vi "FindAllChildrenOf.vi"(10 "Name":string, 11 "RelationshipBrowser":refnum<class "Relationships.lvclass">) -> (3 "Children":refnum<class "Person.lvclass">[](array[class]))   [LabVIEW 2018, in "Relationships.lvclass"]
uses:
  Relationships.lvclass
  Person/Person.lvclass
  Relationships.lvclass/Relationships.ctl
  Person/Person.lvclass/Person.ctl
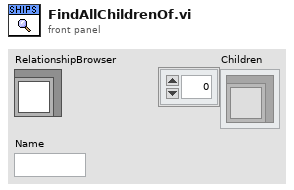
[diagram p1: front panel]
types:
  T1 = typedef "IRelationshipBrowser.lvclass/Relationship.ctl" = enum16{"Sibling", "Child", "Parent"}
  T2 = cluster{"Person A":refnum<class "Person.lvclass">, "Person B":refnum<class "Person.lvclass">, "Relationship A->B":T1}[]
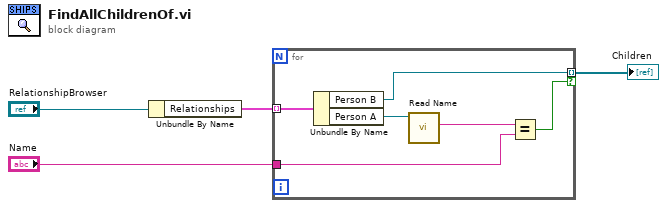
[diagram p0: block diagram]
diagram:
  n1 = Unbundle By Name("RelationshipBrowser") -> ("Relationships"=w3:T2)
  n2 = for {
    tunnel: w3 -> [w10] mode=indexing
    tunnel: [w8] -> w2 mode=indexing if=w5
    tunnel: "Name" -> [w6]
    n3 = Unbundle By Name(w10) -> ("Person B"=w8:refnum<class "Person.lvclass">, "Person A"=w9:refnum<class "Person.lvclass">)
    n4 = call "Read Name.vi"("Person In"=w9) -> ("Name"=w7:string)  [unwired: 9 in, 1 out]
    n5 = Equal?(x=w7, y=w6) -> (x = y?=w5:bool)
  }
  "Children" <- w2
